vi "Read.vi"(8 "error in (no error)":errorcluster, 11 "Numeric Array in":refnum<class "Double Float Array 1D.lvclass">) -> (0 "error out":errorcluster, 2 "Numeric":dbl, 3 "Numeric Array out":refnum<class "Double Float Array 1D.lvclass">)   [LabVIEW 2021, in "Variable.lvlib" / "Double Float Array 1D.lvclass"]
uses:
  Double Float Array 1D.lvclass
  Double Float Array 1D.lvclass/Double Float Array 1D.ctl
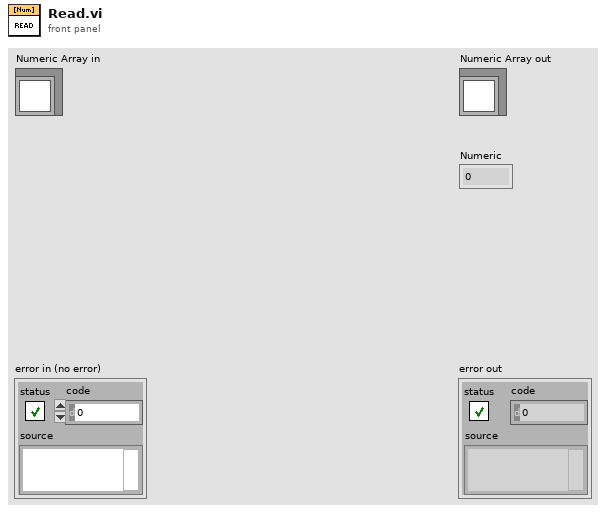
[diagram p1: front panel]
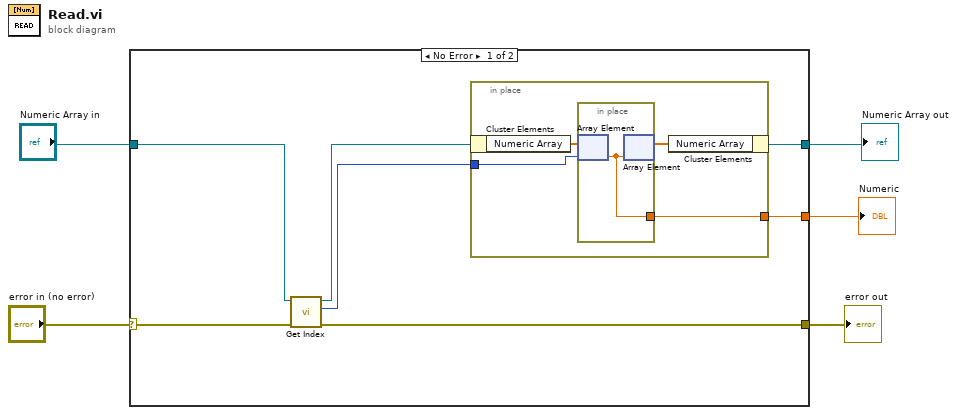
[diagram p0: block diagram]
diagram:
  n1 = case shown="No Error" "error in (no error)" {
    selector: "error in (no error)" -> [w10 w19]
    tunnel: [w9 w19] -> w2
    tunnel: "Numeric Array in" -> [w8 w18]
    tunnel: [w12 w18] -> w4
    tunnel: [w11 _] -> w3
    frame No Error {
      n2 = call-dynamic "Get Index.vi"("error in (no error)"=w10, "Vector Parent in"=w8) -> ("error out"=w9:errorcluster, "Index"=w6:i32, "Vector Parent out"=w7:refnum<class "Double Float Array 1D.lvclass">)  [unwired: 7 in]
      n3 = in-place {
        in-place-border: w6 -> [w15]
        in-place-border: [w13] -> w11
        n4 = in-place-cluster #1(w7) -> ("Numeric Array"=w16:dbl[])
        n5 = in-place {
          in-place-border: [w17] -> w13
          n6 = in-place-array #2(w16, w15) -> (w17:dbl)
          n7 = in-place-array #2(w17) -> (w14:dbl[])  [unwired: 1 out]
        }
        n8 = in-place-cluster #1("Numeric Array"=w14) -> (w12:refnum<class "Double Float Array 1D.lvclass">)
      }
    }
    frame Error {
    }
  }
  "error out" <- w2
  "Numeric Array out" <- w4
  "Numeric" <- w3
